vi "open.local.issue.file.vi"(8 "error in (no error)":errorcluster, 11 "issue json path":path) -> (0 "error out":errorcluster, 3 "issue":T1)   [LabVIEW 2024, in "CV_Shared_Library.lvlib"]
uses:
  CV_Shared_Library.lvlib
  CV_RESTful_Library/typedefs/local_issue--cluster.ctl
  CV_RESTful_Library/typedefs/cv_issue.generic_credit--cluster.ctl
  CV_RESTful_Library/typedefs/cv_issue.associated_image--cluster.ctl
  CV_RESTful_Library/typedefs/cv_issue.person_credit--cluster.ctl
  <vilib>/addons/_JKI.lib/Serialization/JSON/JKI JSON Serialization.lvlib
  CV_RESTful_Library/CV_RESTful_Lib.lvlib
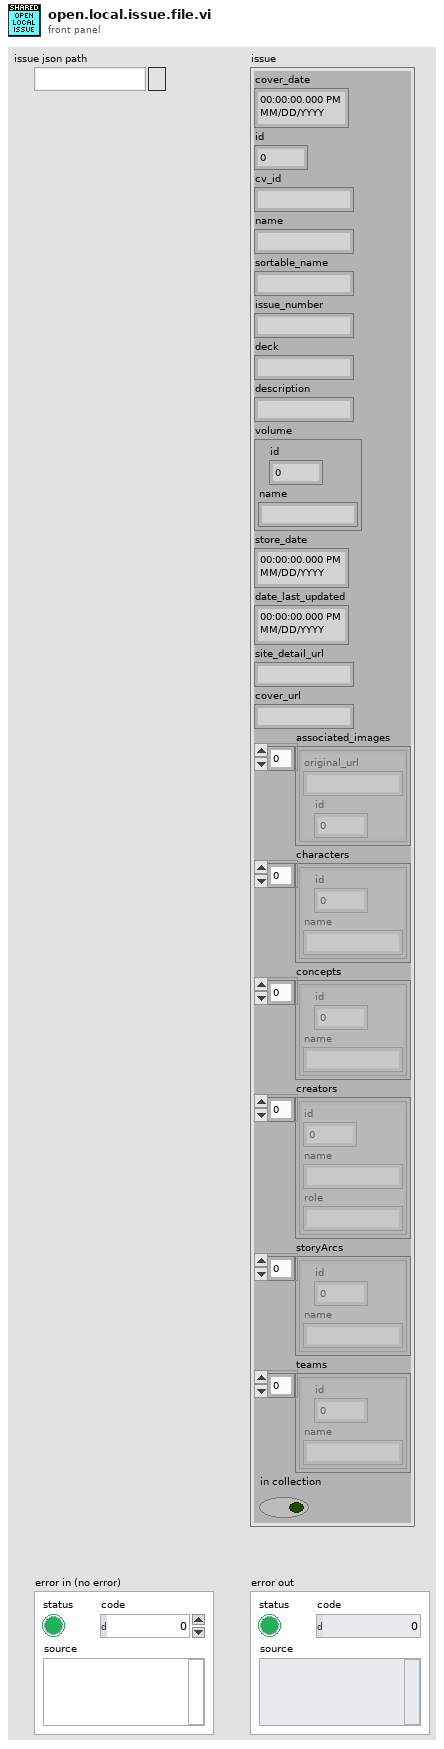
[diagram p1: front panel]
types:
  T1 = typedef "CV_RESTful_Lib.lvlib/local_issue--cluster.ctl" = cluster{"cover_date":timestamp, "id":i32, "cv_id":string, "name":string, "sortable_name":string, "issue_number":string, "deck":string, "description":string, "volume":T2, "store_date":timestamp, "date_last_updated":timestamp, "site_detail_url":string, "cover_url":string, "associated_images":T3[], "characters":T2[], "concepts":T2[], "creators":T4[], "storyArcs":T2[], "teams":T2[], "in collection":bool}
  T2 = typedef "CV_RESTful_Lib.lvlib/cv_issue.generic_credit--cluster.ctl" = cluster{"id":i32, "name":string}
  T3 = typedef "CV_RESTful_Lib.lvlib/cv_issue.associated_image--cluster.ctl" = cluster{"original_url":string, "id":i32}
  T4 = typedef "CV_RESTful_Lib.lvlib/cv_issue.person_credit--cluster.ctl" = cluster{"id":i32, "name":string, "role":string}
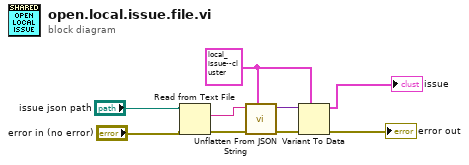
[diagram p0: block diagram]
diagram:
  w6 = T1 {"cover_date"=timestamp(0 s since 1904-01-01), "id"=0, "cv_id"="", "name"="", "sortable_name"="", "issue_number"="", "deck"="", "description"="", "volume"={"id"=0, "name"=""}, "store_date"=timestamp(0 s since 1904-01-01), "date_last_updated"=timestamp(0 s since 1904-01-01), "site_detail_url"="", "cover_url"="", "associated_images"=[], "characters"=[], "concepts"=[], "creators"=[], "storyArcs"=[], "teams"=[], "in collection"=FALSE} ("issue")
  n1 = Read from Text File(file (use dialog)="issue json path", error in="error in (no error)") -> (text=w2:string, error out=w3:errorcluster)  [unwired: 2 in, 2 out]
  n2 = call <vilib>:"Unflatten From JSON String.vi"("Type and Defaults"=w6, "error in"=w3, "JSON String"=w2) -> ("error out"=w4:errorcluster, "Variant"=w5:variant)  [unwired: 7 in]
  n3 = Variant To Data(error in=w4, type=w6, Variant=w5) -> (data=→"issue":T1, error out=→"error out":errorcluster)
